vi "S2C_UNITHERM_Proc_LoadSet.vi"(7 "Local?":bool, 8 "Error In":errorcluster, 10 "Command":string, 11 "JSON String":string) -> (0 "Error Out":errorcluster, 3 "Response":variant)   [LabVIEW 2024]
uses:
  S2C_UNITHERM_Proc_Globals.vi
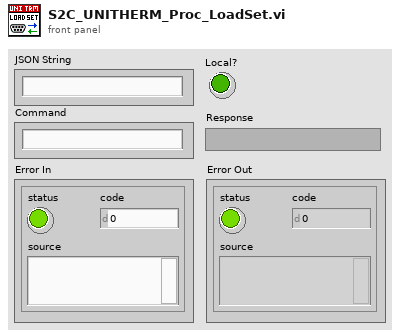
[diagram p1: front panel]
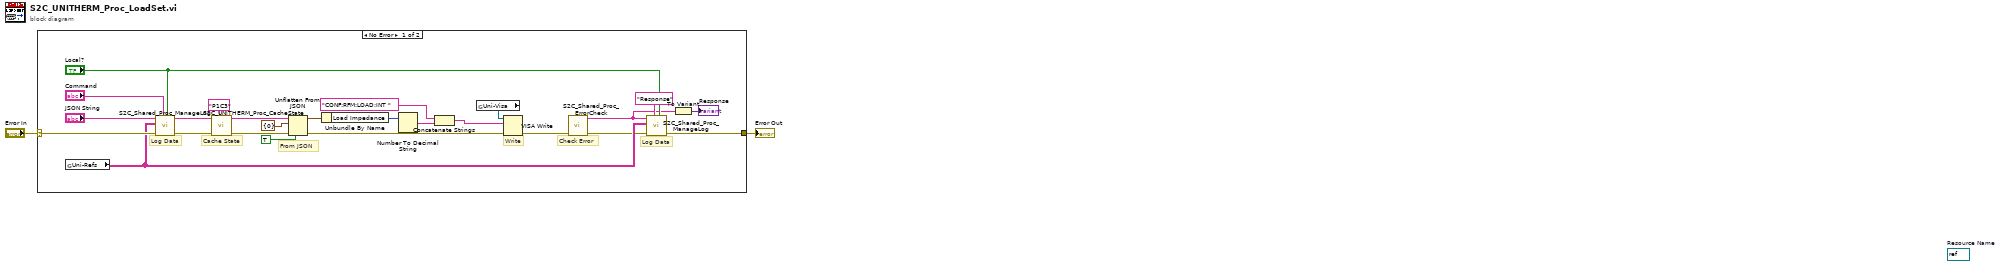
[diagram p0: block diagram]
diagram:
  (unwired) refnum<visa-resource-name> refnum  # Resource Name
  n1 = case shown="No Error" "Error In" {
    selector: "Error In" -> [w23 w28]
    tunnel: [w20 w28] -> w1
    frame No Error {
      # "Check Error"
      # "Cache State"
      # "Write"
      # "Log Data"
      # "Log Data"
      # "From JSON"
      n2 = global read "S2C_UNITHERM_Proc_Globals.vi" "Uni-Refs"() -> (w7:string[][])
      n3 = call "S2C_Shared_Proc_ManageLog.vi"("Local?"="Local?", "Command"="Command", "Error In"=w23, "Refs"=w7, "Data In"="JSON String") -> ("Error Out"=w11:errorcluster, "Data Out"=w10:string)  [unwired: 5 in]
      n4 = call "S2C_UNITHERM_Proc_CacheState.vi"("Label"="P1C3", "Error In"=w11, "Data In"=w10) -> ("Error Out"=w8:errorcluster, "Data Out"=w9:string)  [unwired: 7 in]
      n5 = Unflatten From JSON(JSON string=w9, type and defaults=cluster{"Load Impedance":i32} {"Load Impedance"=0}, default null elements? (F)=TRUE, error in (no error)=w8) -> (value=w26:cluster{"Load Impedance":i32}, error out=w24:errorcluster)  [unwired: 3 in]
      n6 = Unbundle By Name(w26) -> ("Load Impedance"=w16:i32)
      n7 = Number To Decimal String(number=w16) -> (decimal integer string=w14:string)  [unwired: 1 in]
      n8 = Concatenate Strings("CONF:RFM:LOAD:INT ", w14) -> (w13:string)
      n9 = global read "S2C_UNITHERM_Proc_Globals.vi" "Uni-Visa"() -> (w3:refnum<visa-resource-name>)
      n10 = VISA Write(VISA resource name=w3, write buffer=w13, error in (no error)=w24) -> (error out=w6:errorcluster)  [unwired: 2 out]
      n11 = call "S2C_Shared_Proc_ErrorCheck.vi"("Error In"=w6) -> ("Error Out"=w5:errorcluster, "Status"=w4:string)  [unwired: 9 in]
      n12 = call "S2C_Shared_Proc_ManageLog.vi"("Local?"="Local?", "Command"="Response", "Error In"=w5, "Refs"=w7, "Data In"=w4) -> ("Error Out"=w20:errorcluster)  [unwired: 5 in, 1 out]
      n13 = To Variant(anything=w4) -> (Variant=→"Response":variant)
    }
    frame Error {
    }
  }
  "Error Out" <- w1
